vi "Facade 2.vi"(0 "Data In":T5, 2 "Display State In":T2, 3 "Container State":T4) -> (6 "Data Out":T5, 7 "Display State Out":T2, 8 "Action":T1)   [LabVIEW 2011, in "Calendar XControl.xctl"]
uses:
  Calendar XControl.xctl
  Data 2.ctl
  <vilib>/_xctls/Container State.ctl
  State 2.ctl
  Language selection.ctl
  <vilib>/_xctls/Action.ctl
  <vilib>/_xctls/XControlSupport.lvlib
panel:
  in  "Sec ctrl":i32 min=0 max=59 format="%02d"
  in  "Min ctrl":i32 min=0 max=59 format="%02d"
  in  "Hour ctrl":i32 min=0 max=23 format="%02d"
  in  "Year ctrl":i32=2015 min=2000 max=2099 step=1
  in  "Month ctrl":i32(ring)=1 items=["Jan"=1, "Feb"=2, "Mar"=3, "Apr"=4, "May"=5, "Jun"=6, "Jul"=7, "Aug"=8, "Sep"=9, "Oct"=10, "Nov"=11, "Dec"=12]
  out "Calendar ctrl":i32[](listbox)
  # "1. Drop the controls that make up the appearance\nof the XControl here.\n\n2. Resize the window to fit the controls\n\n3. If the XControl is of fixed size,  make the \n window not resizable from VI Properties->Window Appearance.\n\n4. If you want the controls to automatically size when the XControl sizes, check  \"Scale all objects on front panel when window resizes\" in File->VI Properties->Window Size page.\n\n5. Show the block diagram and handle events for the controls on this panel."
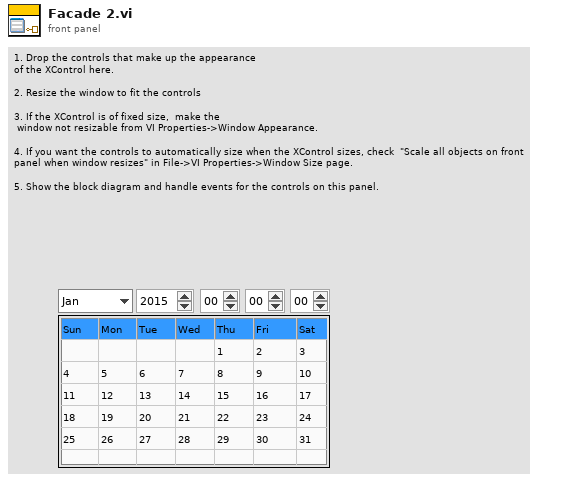
[diagram p1: front panel]
types:
  T1 = typedef "XControlSupport.lvlib/Action.ctl" = cluster{"Data Changed?":bool, "State Changed?":bool, "Action Name":string}
  T2 = typedef "Calendar XControl.xctl/State 2.ctl" = cluster{"Language selection":T3, "Time Stamp":timestamp}
  T3 = typedef "Calendar XControl.xctl/Language selection.ctl" = enum16{"English", "Français", "Español", "Deutsche", "Italiano", "Svenska", "Portugese"}
  T4 = typedef "XControlSupport.lvlib/Container State.ctl" = cluster{"Indicator?":bool, "Run Mode?":bool, " Refnum":refnum<vi>}
  T5 = typedef "Calendar XControl.xctl/Data 2.ctl" = timestamp
  T6 = enum8{"Enabled", "Disabled", "Disabled and Grayed Out"}
  T7 = typedef "LVDateTimeRec.ctl" = cluster{"fractional second":dbl, "second":i32, "minute":i32, "hour":i32, "day of month":i32, "month":i32, "year":i32, "day of week":i32, "day of year":i32, "DST":i32}
  T8 = typedef "LVRowAndColumnTypeDef.ctl" = cluster{"Row":i32, "Column":i32}
  T9 = typedef "LVPoint32TypeDef.ctl" = cluster{"Horizontal":i32, "Vertical":i32}
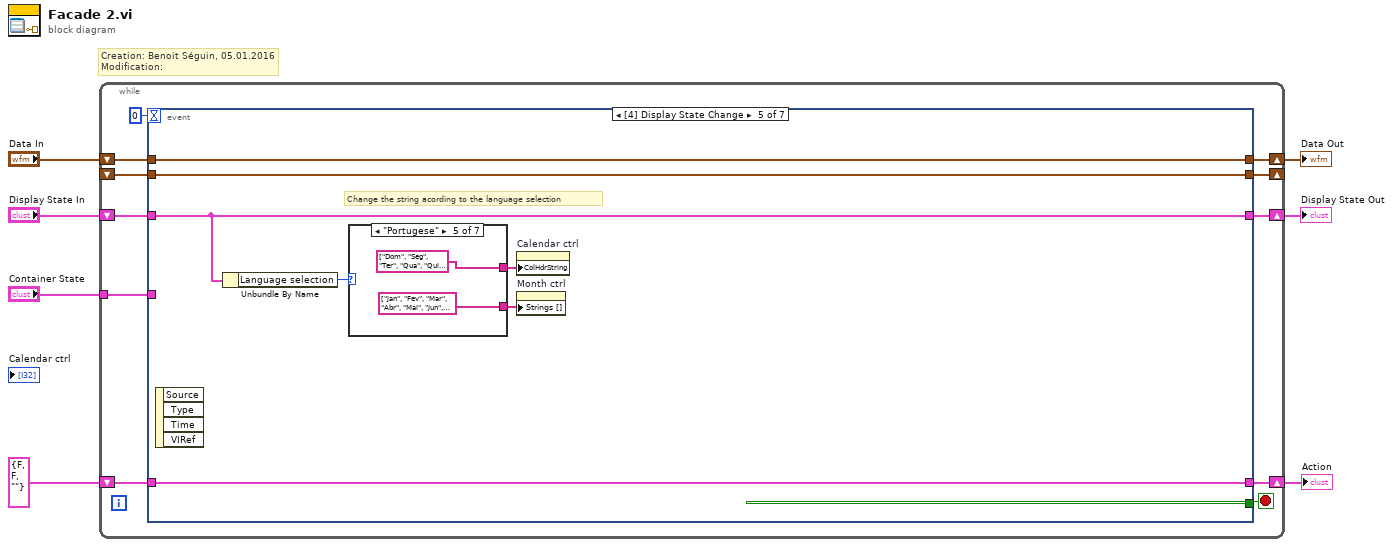
[diagram p0: block diagram]
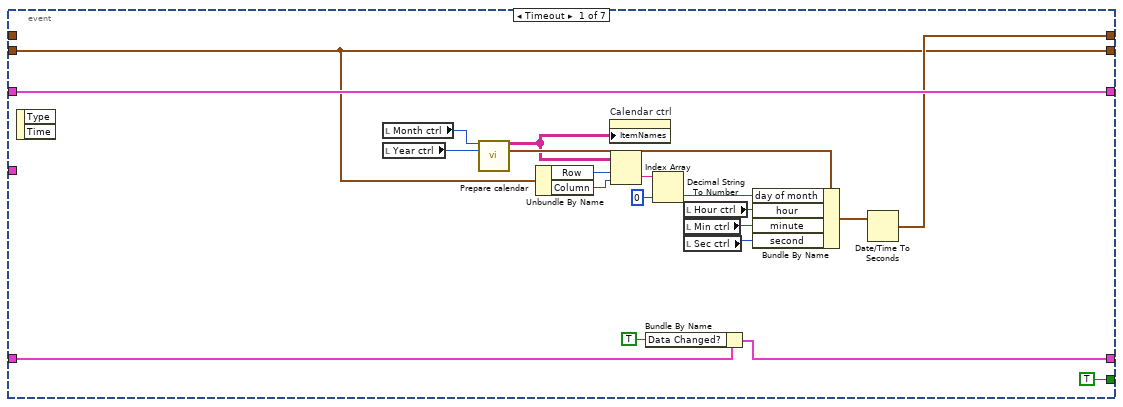
[diagram p2: hidden frame]
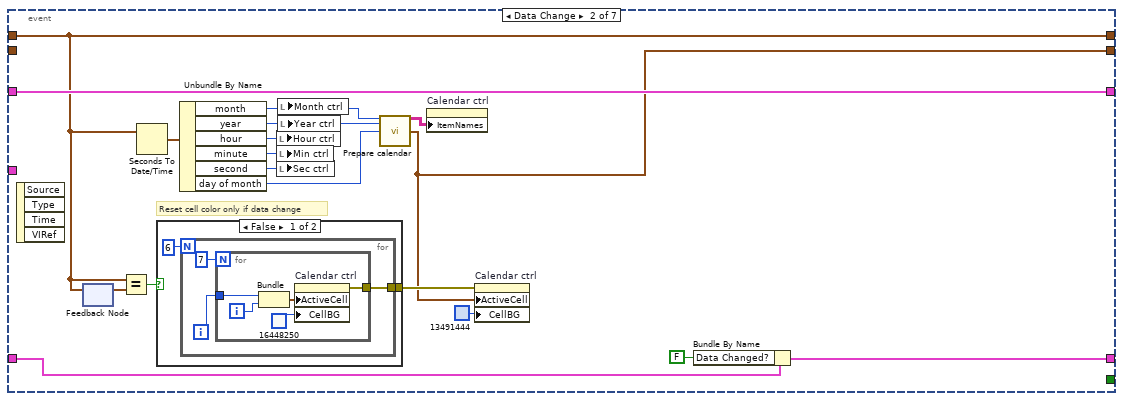
[diagram p3: hidden frame]
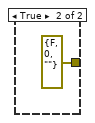
[diagram p4: hidden frame]
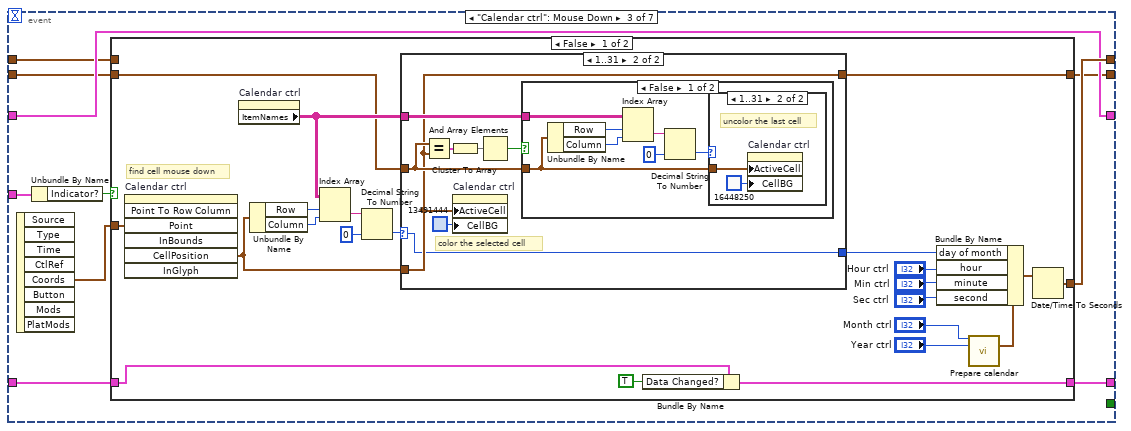
[diagram p5: hidden frame]
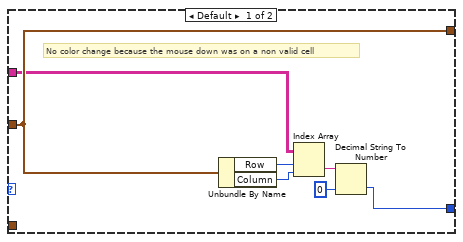
[diagram p6: hidden frame]
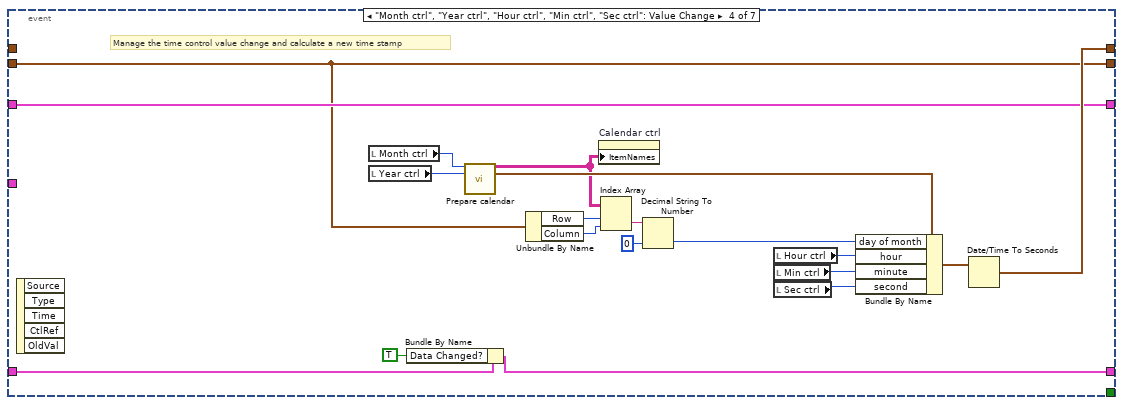
[diagram p10: hidden frame]
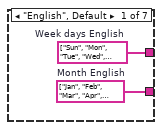
[diagram p11: hidden frame]
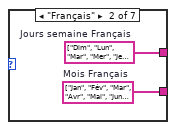
[diagram p12: hidden frame]
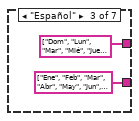
[diagram p13: hidden frame]
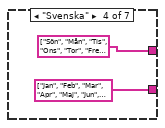
[diagram p14: hidden frame]
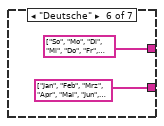
[diagram p15: hidden frame]
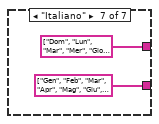
[diagram p16: hidden frame]
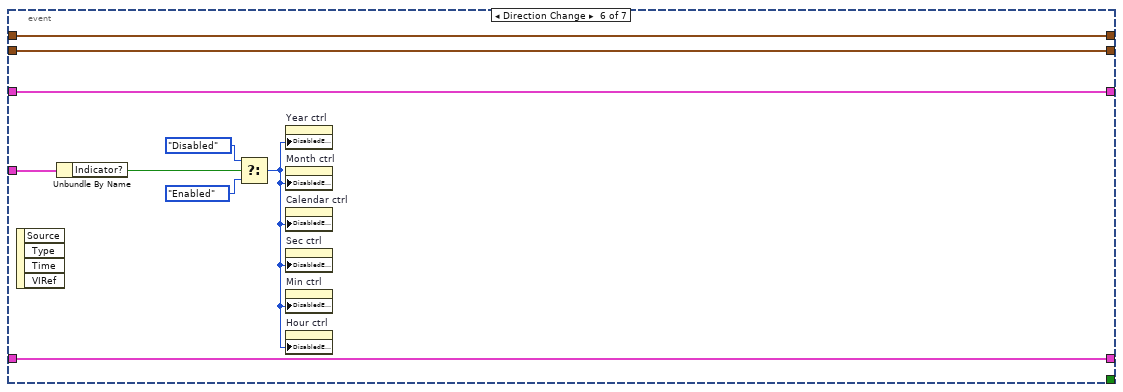
[diagram p17: hidden frame]
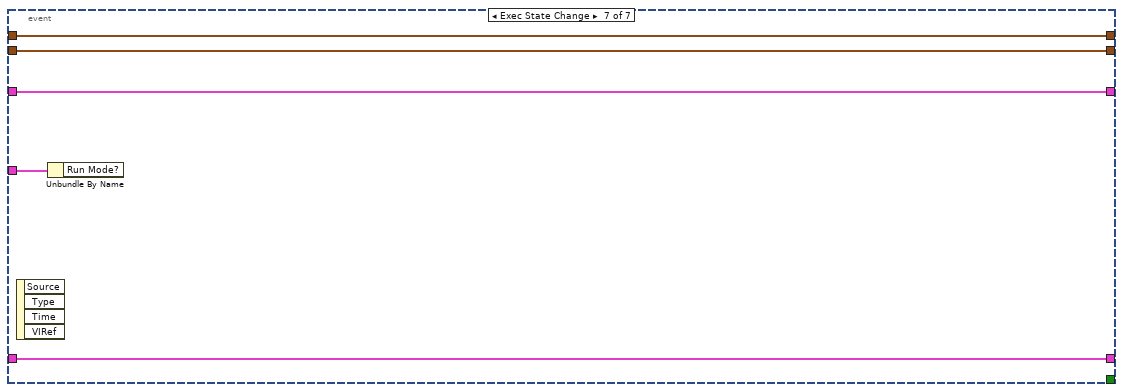
[diagram p18: hidden frame]
diagram:
  # "Creation: Benoit Séguin, 05.01.2016\nModification:"
  n1 = while {
    shift-right: [w17] -> w5
    shift-left: "Display State In" -> [w18]
    tunnel: "Container State" -> [w14]
    shift-right: [w12] -> w1
    shift-left: "Data In" -> [w13]
    shift-right: [w10] -> w3
    shift-left: T1 {"Data Changed?"=FALSE, "State Changed?"=FALSE, "Action Name"=""} ("Action") -> [w11]
    shift-right: [w9] -> _
    shift-left: _ -> [w8]
    stop <- w16 stop-if-true
    n2 = event shown="[4] Display State Change" {
      selector: _ -> [_ _ _ _ _ _ _]
      dyn-events: _ -> [_ _ _ _ _ _ _]
      timeout: 0 -> [_ _ _ _ _ _ _]
      tunnel: w18 -> [w37 w56 w75 w131 w148 w174 w179]
      tunnel: [w37 w56 w75 w131 w148 w174 w179] -> w17
      tunnel: [TRUE _ _ _ _ _ _] -> w16
      tunnel: w14 -> [_ _ w72 _ _ w175 w180]
      tunnel: w13 -> [_ w40 w70 _ w152 w173 w178]
      tunnel: [w23 w40 w77 w142 w152 w173 w178] -> w12
      tunnel: [w21 w53 w68 w128 w151 w172 w177] -> w10
      tunnel: w11 -> [w19 w52 w69 w127 w151 w172 w177]
      tunnel: [w22 w39 w74 w130 w146 w167 w176] -> w9
      tunnel: w8 -> [w22 _ w73 w130 w146 w167 w176]
      event Timeout {
        n3 = event-data() -> ()  [unwired: 1 in, 2 out]
        n4 = local read "Month ctrl"() -> (w33:i32)
        n5 = local read "Year ctrl"() -> (w32:i32)
        n6 = call "Prepare calendar.vi"("Month ctrl"=w33, "Year ctrl"=w32) -> ("Array"=w24:string[][], "date time rec"=w35:T7)  [unwired: 11 in, 1 out]
        n7 = Unbundle By Name(w22) -> ("Row"=w27:i32, "Column"=w28:i32)
        n8 = property on="Calendar ctrl" class="MCListbox (strict)"("ItemNames"=w24) -> ()  [unwired: 2 in, 2 out]
        n9 = Index Array(array=w24, index (row)=w27, index (col)=w28) -> (element=w26:string)
        n10 = Bundle By Name(cluster=w19, "Data Changed?"=TRUE) -> (w21:T1)
        n11 = Decimal String To Number(string=w26, default (0L)=0 ("default (0 I32)")) -> (number=w34:i32)  [unwired: 1 in, 1 out]
        n12 = local read "Hour ctrl"() -> (w29:i32)
        n13 = local read "Min ctrl"() -> (w30:i32)
        n14 = local read "Sec ctrl"() -> (w31:i32)
        n15 = Bundle By Name(cluster=w35, "day of month"=w34, "hour"=w29, "minute"=w30, "second"=w31) -> (w36:T7)
        n16 = Date/Time To Seconds(2:w36) -> (0:w23:timestamp)  [unwired: 1 in]
      }
      event Data Change {
        # "Reset cell color only if data change"
        n17 = event-data() -> ()  [unwired: 1 in, 4 out]
        n18 = feedback-in #1(w40) -> ()
        n19 = feedback #1() -> (w41:T5)  [unwired: 1 in]
        n20 = Equal?(x=w40, y=w41) -> (x = y?=w42:bool)
        n21 = Seconds To Date/Time(time stamp (now)=w40) -> (date time rec=w51:T7)  [unwired: 1 in]
        n22 = case shown="False" w42 {
          tunnel: [w57 errorcluster {"status"=FALSE, "code"=0, "source"=""} ("error out")] -> w43
          frame False {
            n23 = for {
              N: 6 -> [_]
              tunnel: [w59] -> w57
              i -> [w60]
              n24 = for {
                N: 7 -> [_]
                tunnel: w60 -> [w64]
                tunnel: [w65] -> w59
                i -> [w63]
                n25 = Bundle(w64, w63) -> (w66:cluster{i32, i32})  [unwired: 1 in]
                n26 = property on="Calendar ctrl" class="MCListbox (strict)"("ActiveCell"=w66, "CellBG"=u32 16448250) -> (error out=w65:errorcluster)  [unwired: 2 in, 1 out]
              }
            }
          }
          frame True {
          }
        }
        n27 = Unbundle By Name(w51) -> ("month"=w50:i32, "year"=w49:i32, "hour"=w48:i32, "minute"=w47:i32, "second"=w46:i32, "day of month"=w44:i32)
        n28 = local write "Hour ctrl"(w48) -> ()
        n29 = local write "Min ctrl"(w47) -> ()
        n30 = local write "Sec ctrl"(w46) -> ()
        n31 = local write "Month ctrl"(w50) -> ()
        n32 = local write "Year ctrl"(w49) -> ()
        n33 = call "Prepare calendar.vi"("Month ctrl"=w50, "Year ctrl"=w49, "Find day of the month index"=w44) -> ("Array"=w55:string[][], "Day of the month index"=w39:T8)  [unwired: 10 in, 1 out]
        n34 = property on="Calendar ctrl" class="MCListbox (strict)"("ItemNames"=w55) -> ()  [unwired: 2 in, 2 out]
        n35 = property on="Calendar ctrl" class="MCListbox (strict)"(error in=w43, "ActiveCell"=w39, "CellBG"=u32 13491444) -> ()  [unwired: 1 in, 2 out]
        n36 = Bundle By Name(cluster=w52, "Data Changed?"=FALSE) -> (w53:T1)
      }
      event "Calendar ctrl": Mouse Down {
        n37 = event-data() -> ("Coords"=w76:T9)  [unwired: 1 in, 7 out]
        n38 = Unbundle By Name(w72) -> ("Indicator?"=w71:bool)
        n39 = case shown="False" w71 {
          tunnel: [w84 w125] -> w77
          tunnel: w76 -> [w83 _]
          tunnel: [w82 w126] -> w74
          tunnel: w73 -> [w81 w126]
          tunnel: w70 -> [_ w125]
          tunnel: w69 -> [w78 w124]
          tunnel: [w79 w124] -> w68
          frame False {
            # "find cell mouse down"
            n40 = invoke on="Calendar ctrl" class="MCListbox (strict)" method="Point To Row Column"("Point"=w83) -> ("CellPosition"=w93:T8)  [unwired: 6 in, 6 out]
            n41 = property on="Calendar ctrl" class="MCListbox (strict)"() -> ("ItemNames"=w99:string[][])  [unwired: 2 in, 2 out]
            n42 = Unbundle By Name(w93) -> ("Row"=w95:i32, "Column"=w94:i32)
            n43 = Index Array(array=w99, index (row)=w95, index (col)=w94) -> (element=w96:string)
            n44 = Decimal String To Number(string=w96, default (0L)=u8 0 ("default (0 I32)")) -> (number=w98:u8)  [unwired: 1 in, 1 out]
            n45 = case shown="1..31" w98 {
              selector: w98 -> [_ w107]
              tunnel: w81 -> [w102 w113]
              tunnel: w93 -> [_ w108]
              tunnel: w99 -> [w100 w109]
              tunnel: [w102 w108] -> w82
              tunnel: [w101 w107] -> w90
              frame Default {
                # "No color change because the mouse down was on a non valid cell"
                n46 = Unbundle By Name(w102) -> ("Row"=w105:i32, "Column"=w106:i32)
                n47 = Index Array(array=w100, index (row)=w105, index (col)=w106) -> (element=w104:string)
                n48 = Decimal String To Number(string=w104, default (0L)=u8 0 ("default (0 I32)")) -> (number=w101:u8)  [unwired: 1 in, 1 out]
              }
              frame 1..31 {
                # "color the selected cell"
                n49 = Equal?(x=w113, y=w108) -> (x = y?=w112:cluster{"Row":bool, "Column":bool})
                n50 = Cluster To Array(cluster=w112) -> (array=w111:bool[])
                n51 = property on="Calendar ctrl" class="MCListbox (strict)"("ActiveCell"=w108, "CellBG"=u32 13491444) -> ()  [unwired: 2 in, 2 out]
                n52 = And Array Elements(Boolean array=w111) -> (logical AND=w110:bool)
                n53 = case shown="False" w110 {
                  tunnel: w113 -> [w115 _]
                  tunnel: w109 -> [w117 _]
                  frame False {
                    n54 = Unbundle By Name(w115) -> ("Row"=w120:i32, "Column"=w119:i32)
                    n55 = Index Array(array=w117, index (row)=w120, index (col)=w119) -> (element=w118:string)
                    n56 = Decimal String To Number(string=w118, default (0L)=u8 0 ("default (0 I32)")) -> (number=w116:u8)  [unwired: 1 in, 1 out]
                    n57 = case shown="1..31" w116 {
                      tunnel: w115 -> [_ w122]
                      frame 0, Default {
                      }
                      frame 1..31 {
                        # "uncolor the last cell"
                        n58 = property on="Calendar ctrl" class="MCListbox (strict)"("ActiveCell"=w122, "CellBG"=u32 16448250) -> ()  [unwired: 2 in, 2 out]
                      }
                    }
                  }
                  frame True {
                    # "No change on the selected cell"
                  }
                }
              }
            }
            n59 = Bundle By Name(cluster=w78, "Data Changed?"=TRUE) -> (w79:T1)
            n60 = call "Prepare calendar.vi"("Month ctrl"="Month ctrl", "Year ctrl"="Year ctrl") -> ("date time rec"=w91:T7)  [unwired: 11 in, 2 out]
            n61 = Bundle By Name(cluster=w91, "day of month"=w90, "hour"="Hour ctrl", "minute"="Min ctrl", "second"="Sec ctrl") -> (w92:T7)
            n62 = Date/Time To Seconds(2:w92) -> (0:w84:timestamp)  [unwired: 1 in]
          }
          frame True {
            # "In indicator mode, the values are managed in value change event"
          }
        }
      }
      event "Month ctrl", "Year ctrl", "Hour ctrl", "Min ctrl", "Sec ctrl": Value Change {
        # "Manage the time control value change and calculate a new time stamp"
        n63 = event-data() -> ()  [unwired: 1 in, 5 out]
        n64 = local read "Month ctrl"() -> (w141:i32)
        n65 = local read "Year ctrl"() -> (w140:i32)
        n66 = Bundle By Name(cluster=w127, "Data Changed?"=TRUE) -> (w128:T1)
        n67 = call "Prepare calendar.vi"("Month ctrl"=w141, "Year ctrl"=w140) -> ("Array"=w132:string[][], "date time rec"=w144:T7)  [unwired: 11 in, 1 out]
        n68 = Unbundle By Name(w130) -> ("Row"=w135:i32, "Column"=w136:i32)
        n69 = property on="Calendar ctrl" class="MCListbox (strict)"("ItemNames"=w132) -> ()  [unwired: 2 in, 2 out]
        n70 = Index Array(array=w132, index (row)=w135, index (col)=w136) -> (element=w134:string)
        n71 = Decimal String To Number(string=w134, default (0L)=0 ("default (0 I32)")) -> (number=w143:i32)  [unwired: 1 in, 1 out]
        n72 = local read "Hour ctrl"() -> (w137:i32)
        n73 = local read "Min ctrl"() -> (w138:i32)
        n74 = local read "Sec ctrl"() -> (w139:i32)
        n75 = Bundle By Name(cluster=w144, "day of month"=w143, "hour"=w137, "minute"=w138, "second"=w139) -> (w145:T7)
        n76 = Date/Time To Seconds(2:w145) -> (0:w142:timestamp)  [unwired: 1 in]
      }
      event Display State Change {
        # "Change the string acording to the language selection"
        n77 = event-data() -> ()  [unwired: 1 in, 4 out]
        n78 = Unbundle By Name(w148) -> ("Language selection"=w147:T3)
        n79 = case shown="\"Portugese\"" w147 {
          tunnel: [w154 w155 string[] ["Ene", "Feb", "Mar", "Abr", "May", "Jun", "Jul", "Ago", "Sep", "Oct", "Nov", "Dic"] ("Mois Français") string[] ["Jan", "Feb", "Mar", "Apr", "Maj", "Jun", "Jul", "Aug", "Sep", "Okt", "Nov", "Dec"] ("Swedish") string[] ["Jan", "Fev", "Mar", "Abr", "Mai", "Jun", "Jul", "Ago", "Set", "Out", "Nov", "Dez"] ("Portuguese") string[] ["Jan", "Feb", "Mrz", "Apr", "Mai", "Jun", "Jul", "Aug", "Sep", "Okt", "Nov", "Dez"] ("German") string[] ["Gen", "Feb", "Mar", "Apr", "Mag", "Giu", "Lug", "Ago", "Set", "Ott", "Nov", "Dic"] ("Italian")] -> w150
          tunnel: [w153 w156 string[] ["Dom", "Lun", "Mar", "Mié", "Jue", "Vie", "Sáb"] ("Jours semaine Français") string[] ["Sön", "Mån", "Tis", "Ons", "Tor", "Fre", "Lör"] ("Jours semaine Français") string[] ["Dom", "Seg", "Ter", "Qua", "Qui", "Sex", "Sáb"] ("Jours semaine Français") string[] ["So", "Mo", "Di", "Mi", "Do", "Fr", "Sa"] ("German") string[] ["Dom", "Lun", "Mar", "Mer", "Gio", "Ven", "Sab"] ("German")] -> w149
          frame "English", Default {
            w154 = string[] ["Jan", "Feb", "Mar", "Apr", "May", "Jun", "Jul", "Aug", "Sep", "Oct", "Nov", "Dec"]  # Month English
            w153 = string[] ["Sun", "Mon", "Tue", "Wed", "Thu", "Fri", "Sat"]  # Week days English
          }
          frame "Français" {
            w155 = string[] ["Jan", "Fév", "Mar", "Avr", "Mai", "Jun", "Jul", "Aoû", "Sep", "Oct", "Nov", "Déc"]  # Mois Français
            w156 = string[] ["Dim", "Lun", "Mar", "Mer", "Jeu", "Ven", "Sam"]  # Jours semaine Français
          }
          frame "Español" {
          }
          frame "Svenska" {
          }
          frame "Portugese" {
          }
          frame "Deutsche" {
          }
          frame "Italiano" {
          }
        }
        n80 = property on="Calendar ctrl" class="MCListbox (strict)"("ColHdrString"=w149) -> ()  [unwired: 2 in, 2 out]
        n81 = property on="Month ctrl" class="Ring (strict)"("Strings []"=w150) -> ()  [unwired: 2 in, 2 out]
      }
      event Direction Change {
        n82 = event-data() -> ()  [unwired: 1 in, 4 out]
        n83 = Unbundle By Name(w175) -> ("Indicator?"=w168:bool)
        n84 = Select(t=T6."Disabled" ("Disabled"), s=w168, f=T6."Enabled" ("Disabled")) -> (s? t:f=w169:T6)
        n85 = property on="Year ctrl" class="DigNum (strict)"("DisabledEnum"=w169) -> ()  [unwired: 2 in, 2 out]
        n86 = property on="Month ctrl" class="Ring (strict)"("DisabledEnum"=w169) -> ()  [unwired: 2 in, 2 out]
        n87 = property on="Calendar ctrl" class="MCListbox (strict)"("DisabledEnum"=w169) -> ()  [unwired: 2 in, 2 out]
        n88 = property on="Sec ctrl" class="DigNum (strict)"("DisabledEnum"=w169) -> ()  [unwired: 2 in, 2 out]
        n89 = property on="Min ctrl" class="DigNum (strict)"("DisabledEnum"=w169) -> ()  [unwired: 2 in, 2 out]
        n90 = property on="Hour ctrl" class="DigNum (strict)"("DisabledEnum"=w169) -> ()  [unwired: 2 in, 2 out]
      }
      event Exec State Change {
        n91 = event-data() -> ()  [unwired: 1 in, 4 out]
        n92 = Unbundle By Name(w180) -> ()  [unwired: 1 out]
      }
    }
  }
  "Display State Out" <- w5
  "Data Out" <- w1
  "Action" <- w3
